vi "niRFUtil MASMT Linear Fit (DBL).vi"(0 "Y":dbl[](array[numeric]), 1 "method":i32(ring) items=["Least Square", "Least Absolute Residual", "Bisquare"], 5 "X":dbl[](array[numeric]), 7 "Weight":dbl[](array[numeric]), 9 "tolerance":dbl=9.999999747378752e-05, 11 "error in (no error)":errorcluster, 12 "parameter bounds":T1={"slope min"=-inf, "slope max"=inf, "intercept min"=-inf, "intercept max"=inf}) -> (4 "Best Linear Fit":dbl[](array[numeric]), 6 "slope":dbl, 8 "intercept":dbl, 10 "residue":dbl, 15 "error out":errorcluster)   [LabVIEW 2015, in "niRFUtil.lvlib"]
doc: "Returns the linear fit of a data set (<B>X</B>, <B>Y</B>) using the Least Square, Least Absolute Residual, or Bisquare method."
uses:
  niRFUtil.lvlib
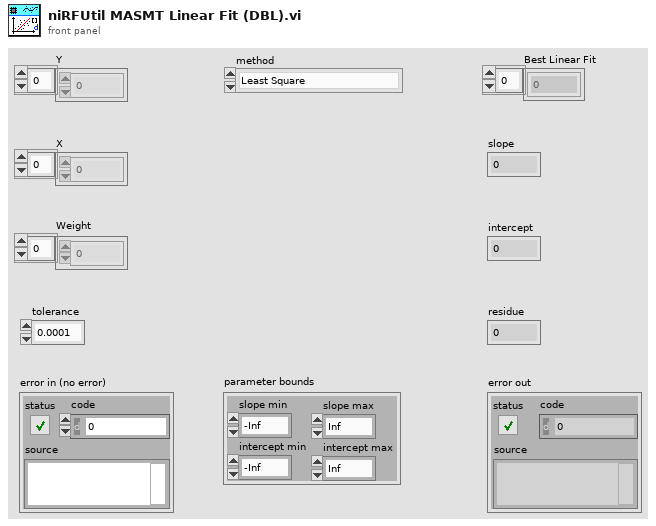
[diagram p1: front panel]
types:
  T1 = cluster{"slope min":dbl, "slope max":dbl, "intercept min":dbl, "intercept max":dbl}
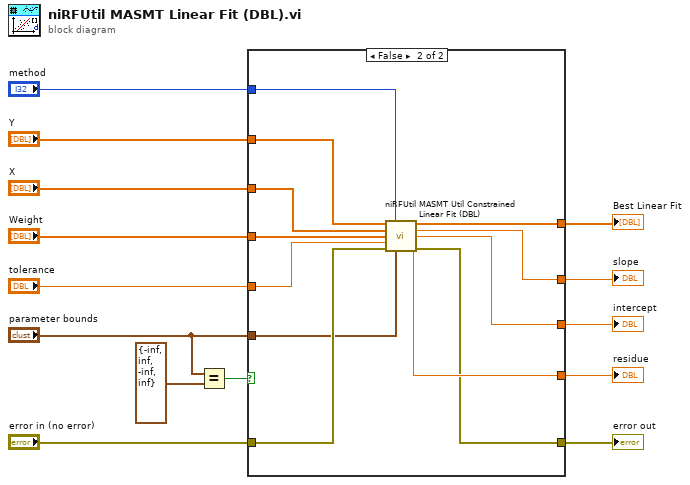
[diagram p0: block diagram]
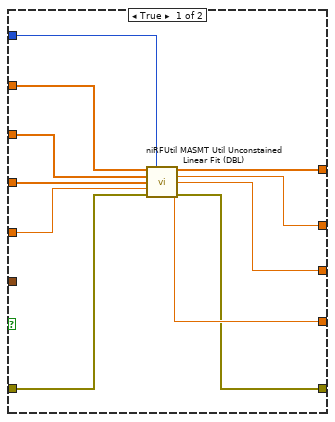
[diagram p2: hidden frame]
diagram:
  n1 = Equal?(x="parameter bounds", y=T1 {"slope min"=-inf, "slope max"=inf, "intercept min"=-inf, "intercept max"=inf} ("parameter bounds")) -> (x = y?=w6:bool)
  n2 = case shown="False" w6 {
    tunnel: "Y" -> [w25 w37]
    tunnel: "X" -> [w24 w36]
    tunnel: "Weight" -> [w23 w35]
    tunnel: "tolerance" -> [w21 w33]
    tunnel: [w17 w29] -> w13
    tunnel: [w18 w30] -> w12
    tunnel: [w19 w31] -> w11
    tunnel: [w20 w32] -> w10
    tunnel: "method" -> [w22 w34]
    tunnel: "parameter bounds" -> [_ w26]
    tunnel: "error in (no error)" -> [w16 w28]
    tunnel: [w15 w27] -> w1
    frame True {
      n3 = call "niRFUtil MASMT Util Unconstained Linear Fit (DBL).vi"("Y"=w25, "method"=w22, "X"=w24, "Weight"=w23, "tolerance"=w21, "error in (no error)"=w16) -> ("Best Linear Fit"=w17:dbl[], "slope"=w18:dbl, "intercept"=w19:dbl, "residue"=w20:dbl, "error out"=w15:errorcluster)  [unwired: 5 in]
    }
    frame False {
      n4 = call "niRFUtil MASMT Util Constrained Linear Fit (DBL).vi"("Y"=w37, "method"=w34, "X"=w36, "Weight"=w35, "tolerance"=w33, "error in (no error)"=w28, "parameter bounds"=w26) -> ("Best Linear Fit"=w29:dbl[], "slope"=w30:dbl, "intercept"=w31:dbl, "residue"=w32:dbl, "error out"=w27:errorcluster)  [unwired: 4 in]
    }
  }
  "intercept" <- w11
  "slope" <- w12
  "Best Linear Fit" <- w13
  "residue" <- w10
  "error out" <- w1
